vi "Test.vi"() -> ()   [LabVIEW 2017]
uses:
  <vilib>/Skyline/Tag/Shared/typedefs/TagProperty.ctl
  <vilib>/Skyline/Tag/Wrapper/Wrapper AMQP_class/Query Tags AMQP.vi
  <vilib>/Skyline/Tag/Wrapper/Wrapper_class/Close Tag (Multiple).vi
  <vilib>/Skyline/Tag/Wrapper/Wrapper_class/NI Skyline Tag.lvclass
  <vilib>/Skyline/Tag/Wrapper/Wrapper AMQP_class/NI Skyline Tag AMQP.lvclass
  <vilib>/Skyline/Tag/Shared/NI Skyline Tag.lvlib
panel:
  out "Numeric":i32
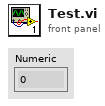
[diagram p1: front panel]
types:
  T1 = typedef "NI Skyline Tag.lvlib/TagProperty.ctl" = cluster{"key":string, "value":string}
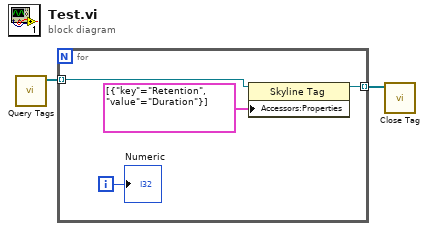
[diagram p0: block diagram]
diagram:
  n1 = call-poly <vilib>:"Query Tags.vi"() -> ("tags"=w2:refnum<class "NI Skyline Tag.lvclass">[])  [unwired: 9 in, 2 out]
  n2 = for {
    tunnel: w2 -> [w4] mode=indexing
    tunnel: [w3] -> w1 mode=indexing
    i -> [w6]
    n3 = property on="Property Node" class="Skyline Tag"(reference=w4, "Accessors:Properties"=T1[] [{"key"="Retention", "value"="Duration"}] ("Properties")) -> (reference out=w3:refnum<class "NI Skyline Tag.lvclass">)  [unwired: 1 in, 1 out]
    "Numeric" <- w6
  }
  n4 = call-poly <vilib>:"Close Tag.vi"("tags in"=w1) -> ()  [unwired: 10 in, 1 out]
